vi "DetectHardware.vi"(8 "error in (no error)":errorcluster, 11 "DemoMicrosope in":refnum<class "DemoMicrosope.lvclass">) -> (0 "error out":errorcluster, 3 "DemoMicrosope out":refnum<class "DemoMicrosope.lvclass">)   [LabVIEW 2020, in "DemoMicrosope.lvlib" / "DemoMicrosope.lvclass"]
uses:
  DemoMicrosope.lvclass
  E:/Development/DevHardSoftware/MicroscopyFramework/Model/Hardware Abstraction Layer/Microscope/Microscope/Microscope.lvclass
  DemoStage/DemoStage/DemoStage.lvclass
  E:/Development/DevHardSoftware/MicroscopyFramework/Model/Hardware Abstraction Layer/Component/Device/Device/Device.lvclass
  DemoStepMotor/DemoStepMotor/DemoStepMotor.lvclass
  DemoDAQ/DemoDAQ/DemoDAQ.lvclass
  DemoCamera/DemoCamera/DemoCamera.lvclass
  DemoLasers/DemoLasers/DemoLasers.lvclass
  Hardware Abstraction Layer/Microscope/Microscope/Microscope.lvclass
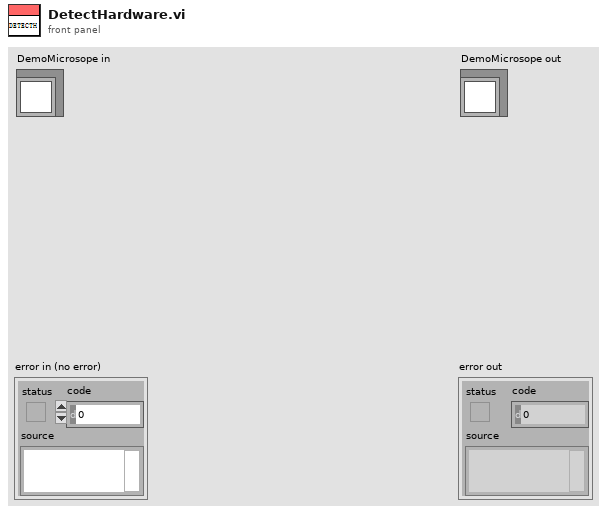
[diagram p1: front panel]
types:
  T1 = cluster{"Label":string, "DeviceType":string, "DefaultDevice? (F)":bool, "StartAcquiring? (F)":bool}
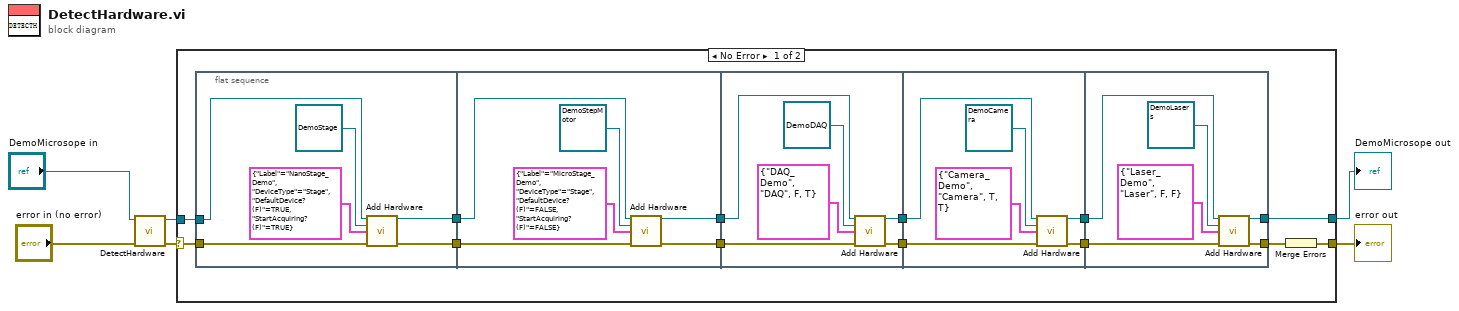
[diagram p0: block diagram]
diagram:
  n1 = call-parent "DetectHardware.vi"("error in (no error)"="error in (no error)", "Microscope in"="DemoMicrosope in") -> ("error out"=w3:errorcluster, "Microscope out"=w4:refnum<class "DemoMicrosope.lvclass">)  [unwired: 8 in]
  n2 = case shown="No Error" w3 {
    selector: w3 -> [w16 w51]
    tunnel: [w17 w51] -> w1
    tunnel: [w18 w50] -> w2
    tunnel: w4 -> [w7 w50]
    frame No Error {
      n3 = flat-sequence {
        tunnel: [w23] -> w19
        tunnel: w16 -> [w25]
        tunnel: [w24] -> w14
        tunnel: w7 -> [w22]
        tunnel: w19 -> [w31]
        tunnel: [w30] -> w15
        tunnel: w14 -> [w29]
        tunnel: [w28] -> w13
        tunnel: w15 -> [w37]
        tunnel: w13 -> [w35]
        tunnel: [w36] -> w12
        tunnel: [w34] -> w10
        tunnel: w12 -> [w43]
        tunnel: [w40] -> w11
        tunnel: w10 -> [w42]
        tunnel: [w41] -> w9
        tunnel: [w48] -> w18
        tunnel: w11 -> [w49]
        tunnel: w9 -> [w47]
        tunnel: [w46] -> w8
        frame #0 {
          n4 = call "Add Hardware.vi"("Microscope in"=w22, "Device.lvlib:Device.lvclass"=refnum<class "DemoStage.lvclass"> refnum ("DemoStage.lvlib:DemoStage.lvclass"), "Setting"=T1 {"Label"="NanoStage_Demo", "DeviceType"="Stage", "DefaultDevice? (F)"=TRUE, "StartAcquiring? (F)"=TRUE}, "error in (no error)"=w25) -> ("Microscope out"=w23:refnum<class "DemoMicrosope.lvclass">, "error out"=w24:errorcluster)  [unwired: 8 in, 2 out]
        }
        frame #1 {
          n5 = call "Add Hardware.vi"("Microscope in"=w31, "Device.lvlib:Device.lvclass"=refnum<class "DemoStepMotor.lvclass"> refnum ("DemoStepMotor.lvlib:DemoStepMotor.lvclass"), "Setting"=T1 {"Label"="MicroStage_Demo", "DeviceType"="Stage", "DefaultDevice? (F)"=FALSE, "StartAcquiring? (F)"=FALSE}, "error in (no error)"=w29) -> ("Microscope out"=w30:refnum<class "DemoMicrosope.lvclass">, "error out"=w28:errorcluster)  [unwired: 8 in, 2 out]
        }
        frame #2 {
          n6 = call "Add Hardware.vi"("Microscope in"=w37, "Device.lvlib:Device.lvclass"=refnum<class "DemoDAQ.lvclass"> refnum ("DemoDAQ.lvlib:DemoDAQ.lvclass"), "Setting"=T1 {"Label"="DAQ_Demo", "DeviceType"="DAQ", "DefaultDevice? (F)"=FALSE, "StartAcquiring? (F)"=TRUE}, "error in (no error)"=w35) -> ("Microscope out"=w36:refnum<class "DemoMicrosope.lvclass">, "error out"=w34:errorcluster)  [unwired: 8 in, 2 out]
        }
        frame #3 {
          n7 = call "Add Hardware.vi"("Microscope in"=w43, "Device.lvlib:Device.lvclass"=refnum<class "DemoCamera.lvclass"> refnum ("DemoCamera.lvlib:DemoCamera.lvclass"), "Setting"=T1 {"Label"="Camera_Demo", "DeviceType"="Camera", "DefaultDevice? (F)"=TRUE, "StartAcquiring? (F)"=TRUE}, "error in (no error)"=w42) -> ("Microscope out"=w40:refnum<class "DemoMicrosope.lvclass">, "error out"=w41:errorcluster)  [unwired: 8 in, 2 out]
        }
        frame #4 {
          n8 = call "Add Hardware.vi"("Microscope in"=w49, "Device.lvlib:Device.lvclass"=refnum<class "DemoLasers.lvclass"> refnum ("DemoLasers.lvlib:DemoLasers.lvclass"), "Setting"=T1 {"Label"="Laser_Demo", "DeviceType"="Laser", "DefaultDevice? (F)"=FALSE, "StartAcquiring? (F)"=FALSE}, "error in (no error)"=w47) -> ("Microscope out"=w48:refnum<class "DemoMicrosope.lvclass">, "error out"=w46:errorcluster)  [unwired: 8 in, 2 out]
        }
      }
      n9 = Merge Errors(w8) -> (w17:errorcluster)
    }
    frame Error {
    }
  }
  "error out" <- w1
  "DemoMicrosope out" <- w2
